vi "Lidar_Main_Tim551.vi"() -> ()   [LabVIEW 2015]
uses:
  <vilib>/Utility/error.llb/DialogType.ctl
panel:
  out "LidarSteers":T1
  out "ROI data":cluster{"배열":bool[]}
  out "AEB":bool
  in  "정지 버튼":bool
  out "전체":cluster{cluster{"x":dbl, "y":dbl}[]}[](graph)
  out "회피범위":cluster{cluster{"x":dbl, "y":dbl}[]}[](graph)
  out "xy 1d clust":cluster{"x":dbl, "y":dbl}[](array[cluster])
  out "frame rate(Hz)":u32=11
  # "Lidar"
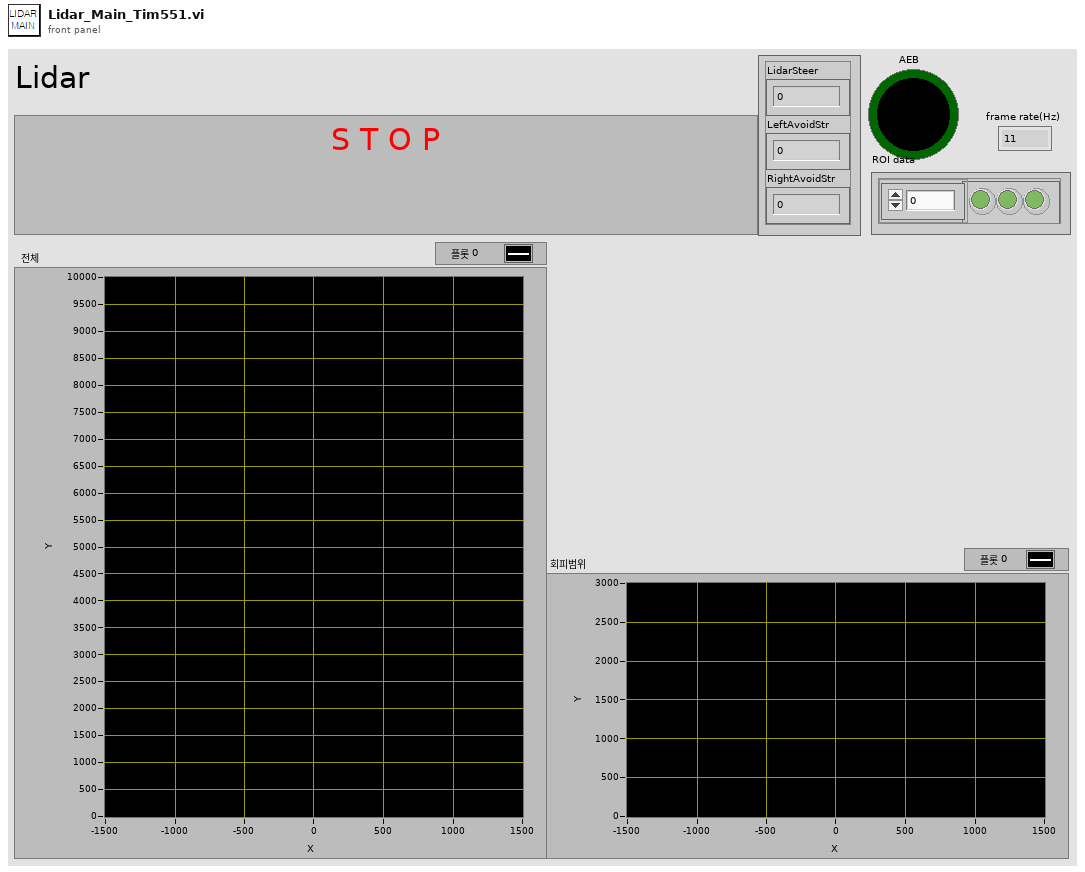
[diagram p1: front panel]
types:
  T1 = cluster{"LidarSteer":dbl, "LeftAvoidStr":dbl, "RightAvoidStr":dbl}
  T2 = enum16{"Standard", "Buffered", "CRLF", "Immediate"}
  T3 = typedef "DialogType.ctl" = u16
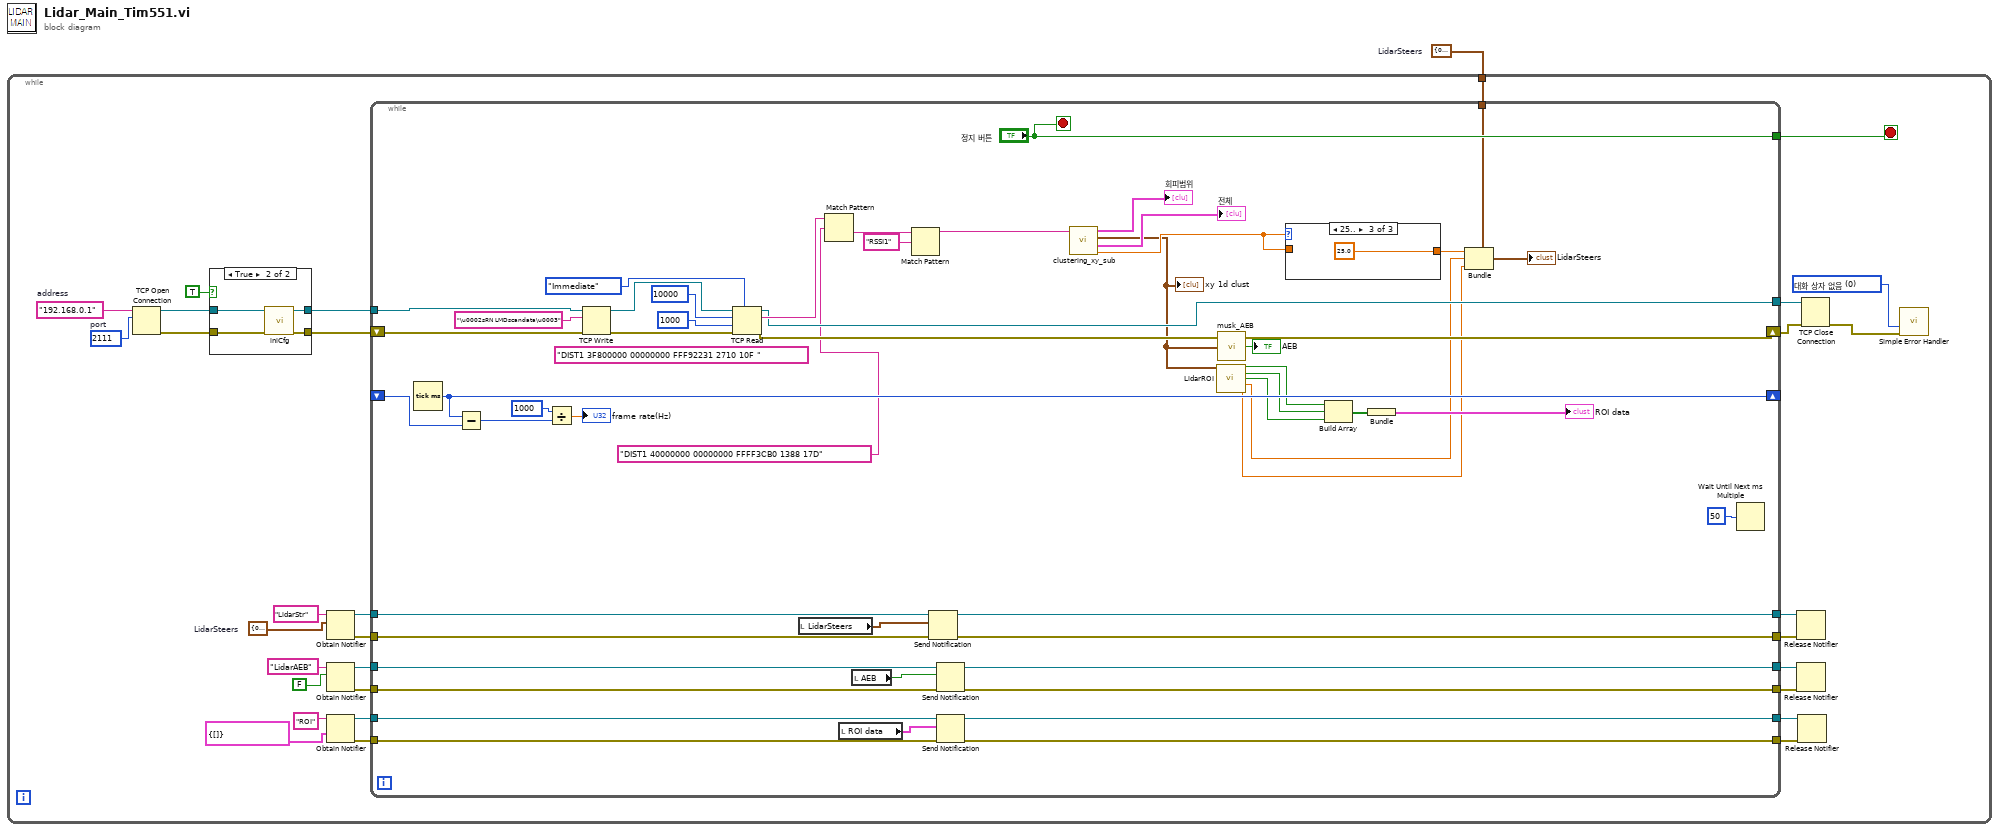
[diagram p0: block diagram]
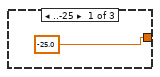
[diagram p2: hidden frame]
diagram:
  w1 = T1 {"LidarSteer"=0.0, "LeftAvoidStr"=0.0, "RightAvoidStr"=0.0}  # LidarSteers
  n1 = while {
    tunnel: w1 -> [w15]
    stop <- w22 stop-if-true
    w14 = T1 {"LidarSteer"=0.0, "LeftAvoidStr"=0.0, "RightAvoidStr"=0.0}  # LidarSteers
    w25 = T3 0 items=["대화 상자 없음", "확인 메시지", "메시지 지속 또는 정지", "확인 메시지 + 경고", "지속/정지 + 경고"] ("type of dialog (OK msg:1)")
    w29 = u16 2111  # port
    w30 = "192.168.0.1"  # address
    n2 = TCP Open Connection(address=w30, remote port or service name=w29) -> (connection ID=w28:refnum<k5>, error out=w27:errorcluster)  [unwired: 3 in]
    n3 = case shown="True" TRUE {
      tunnel: w28 -> [w89 w93]
      tunnel: w27 -> [w88 w92]
      tunnel: [w89 w91] -> w32
      tunnel: [w88 w90] -> w31
      frame False {
      }
      frame True {
        n4 = call "iniCfg.vi"("error out"=w92, "connection ID"=w93) -> ("error out 2"=w90:errorcluster, "connection ID 2"=w91:refnum<k5>)  [unwired: 8 in]
      }
    }
    n5 = Obtain Notifier(name (unnamed)="LidarStr" ("이름(이름없음)"), notification data type=w14) -> (notifier out=w13:refnum<notifier>, error out=w2:errorcluster)  [unwired: 2 in, 1 out]
    n6 = Obtain Notifier(name (unnamed)="LidarAEB" ("이름(이름없음)"), notification data type=FALSE) -> (notifier out=w3:refnum<notifier>, error out=w4:errorcluster)  [unwired: 2 in, 1 out]
    n7 = Obtain Notifier(name (unnamed)="ROI" ("이름(이름없음)"), notification data type=cluster{bool[]} {[]}) -> (notifier out=w5:refnum<notifier>, error out=w6:errorcluster)  [unwired: 2 in, 1 out]
    n8 = while {
      tunnel: w32 -> [w77]
      shift-right: [w82] -> w23
      shift-left: w31 -> [w73]
      shift-right: [w71] -> _
      shift-left: _ -> [w72]
      tunnel: ["정지 버튼"] -> w22
      tunnel: [w63] -> w21
      tunnel: w15 -> [w39]
      tunnel: w13 -> [w51]
      tunnel: [w50] -> w12
      tunnel: [w49] -> w11
      tunnel: [w48] -> w10
      tunnel: [w47] -> w9
      tunnel: [w46] -> w8
      tunnel: [w45] -> w7
      tunnel: w6 -> [w44]
      tunnel: w5 -> [w43]
      tunnel: w4 -> [w42]
      tunnel: w3 -> [w41]
      tunnel: w2 -> [w40]
      stop <- "정지 버튼" stop-if-true
      (unwired) "DIST1 3F800000 00000000 FFF92231 2710 10F " ("정규식")
      n9 = Tick Count (ms)() -> (millisecond timer value=w71:u32)
      n10 = Subtract(x=w71, y=w72) -> (x-y=w70:u32)
      n11 = Divide(x=u32 1000, y=w70) -> (x/y=→"frame rate(Hz)":dbl)
      n12 = TCP Write(connection ID=w77, data in="\u0002sRN LMDscandata\u0003", error in (no error)=w73) -> (connection ID out=w84:refnum<k5>, error out=w78:errorcluster)  [unwired: 1 in, 1 out]
      n13 = TCP Read(connection ID=w84, bytes to read=10000 ("읽을 바이트"), error in (no error)=w78, 7:T2."Immediate" ("모드(standard)"), 9:1000 ("타임아웃 ms (25000)")) -> (connection ID out=w63:refnum<k5>, data out=w74:string, error out=w82:errorcluster)
      n14 = local read "LidarSteers"() -> (w34:T1)
      n15 = Match Pattern(string=w74, regular expression="DIST1 40000000 00000000 FFFF3CB0 1388 17D" ("정규식")) -> (after substring=w76:string)  [unwired: 1 in, 3 out]
      n16 = local read "ROI data"() -> (w53:cluster{"배열":bool[]})
      n17 = local read "AEB"() -> (w52:bool)
      n18 = Match Pattern(string=w76, regular expression="RSSI1" ("정규식")) -> (before substring=w65:string)  [unwired: 1 in, 3 out]
      n19 = Send Notification(notification=w34, notifier=w51, error in (no error)=w40) -> (notifier out=w50:refnum<notifier>, error out=w49:errorcluster)
      n20 = Send Notification(notification=w52, notifier=w41, error in (no error)=w42) -> (notifier out=w48:refnum<notifier>, error out=w47:errorcluster)
      n21 = Send Notification(notification=w53, notifier=w43, error in (no error)=w44) -> (notifier out=w46:refnum<notifier>, error out=w45:errorcluster)
      n22 = call "clustering_xy_sub.vi"("r값 문자열"=w65) -> ("steer"=w62:dbl, "전체 관찰용"=→"전체":cluster{cluster{"x":dbl, "y":dbl}[]}[], "xy 1d clust"=w59:cluster{"x":dbl, "y":dbl}[], "주행 관찰용"=→"회피범위":cluster{cluster{"x":dbl, "y":dbl}[]}[])  [unwired: 7 in]
      "xy 1d clust" <- w59
      n23 = call "LidarROI.vi"("x,y 배열"=w59) -> ("ROI1"=w58:bool, "ROI2"=w57:bool, "ROI3"=w56:bool, "왼쪽정적라이다스티어"=w37:dbl, "오른쪽정적라이다스티어"=w36:dbl)  [unwired: 10 in]
      n24 = call "musk_AEB.vi"("x,y 배열"=w59) -> ("AEB!!"=→"AEB":bool)
      n25 = case shown="25.." w62 {
        tunnel: [-25.0 w86 25.0] -> w38
        tunnel: w62 -> [_ w86 _]
        frame ..-25 {
        }
        frame 0, Default {
        }
        frame 25.. {
        }
      }
      n26 = Build Array(w58, w57, w56) -> (w55:bool[])
      n27 = Bundle(w55) -> (→"ROI data":cluster{bool[]})  [unwired: 1 in]
      n28 = Bundle(cluster=w39, "LidarSteer"=w38, "LeftAvoidStr"=w37, "RightAvoidStr"=w36) -> (→"LidarSteers":T1)
      n29 = Wait Until Next ms Multiple(millisecond multiple=u32 50 ("ms 배수")) -> ()  [unwired: 1 out]
    }
    n30 = Release Notifier(notifier=w12, error in (no error)=w11) -> ()  [unwired: 1 in, 3 out]
    n31 = Release Notifier(notifier=w10, error in (no error)=w9) -> ()  [unwired: 1 in, 3 out]
    n32 = Release Notifier(notifier=w8, error in (no error)=w7) -> ()  [unwired: 1 in, 3 out]
    n33 = TCP Close Connection(connection ID=w21, error in (no error)=w23) -> (error out=w24:errorcluster)  [unwired: 1 in, 1 out]
    n34 = call <vilib>:"Simple Error Handler.vi"("type of dialog (OK msg:1)"=w25, "error in (no error)"=w24) -> ()  [unwired: 3 in, 5 out]
  }
